vi "Edwin_VI01.vi"(8 "VC":dbl, 11 "VE":dbl[](array[numeric])) -> (3 "VF":dbl)   [LabVIEW 2018]
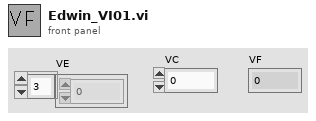
[diagram p1: front panel]
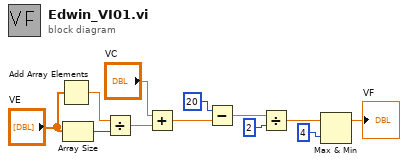
[diagram p0: block diagram]
diagram:
  n1 = Add Array Elements(numeric array="VE") -> (sum=w10:dbl)
  n2 = Array Size(array="VE") -> (size(s)=w9:i32)
  n3 = Divide(x=w10, y=w9) -> (x/y=w8:dbl)
  n4 = Add(x="VC", y=w8) -> (x+y=w6:dbl)
  n5 = Subtract(x=20, y=w6) -> (x-y=w4:dbl)
  n6 = Divide(x=w4, y=2) -> (x/y=w2:dbl)
  n7 = Max & Min(x=w2, y=4) -> (max(x,y)=→"VF":dbl)  [unwired: 1 out]
